vi "Peak tracking sq.vi"(4 "BF len":i32, 6 "EnH choice":u16(ring) items=["Off", "Linear best fit"], 7 "Error control":sgl, 8 "Trace":i32=1, 9 "Poly count":i32=4, 10 "Int IN":sgl[](array[numeric]), 11 "Scan":sgl[][](array[numeric])) -> (2 "Int Out":sgl[](array[numeric]), 3 "Scan Out":sgl[](array[numeric]))   [LabVIEW 2014]
uses:
  <vilib>/Analysis/NI_AALPro.lvlib
panel:
  out "Locations":sgl[](array[numeric])
  # "See block diagram"
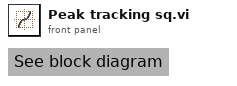
[diagram p1: front panel]
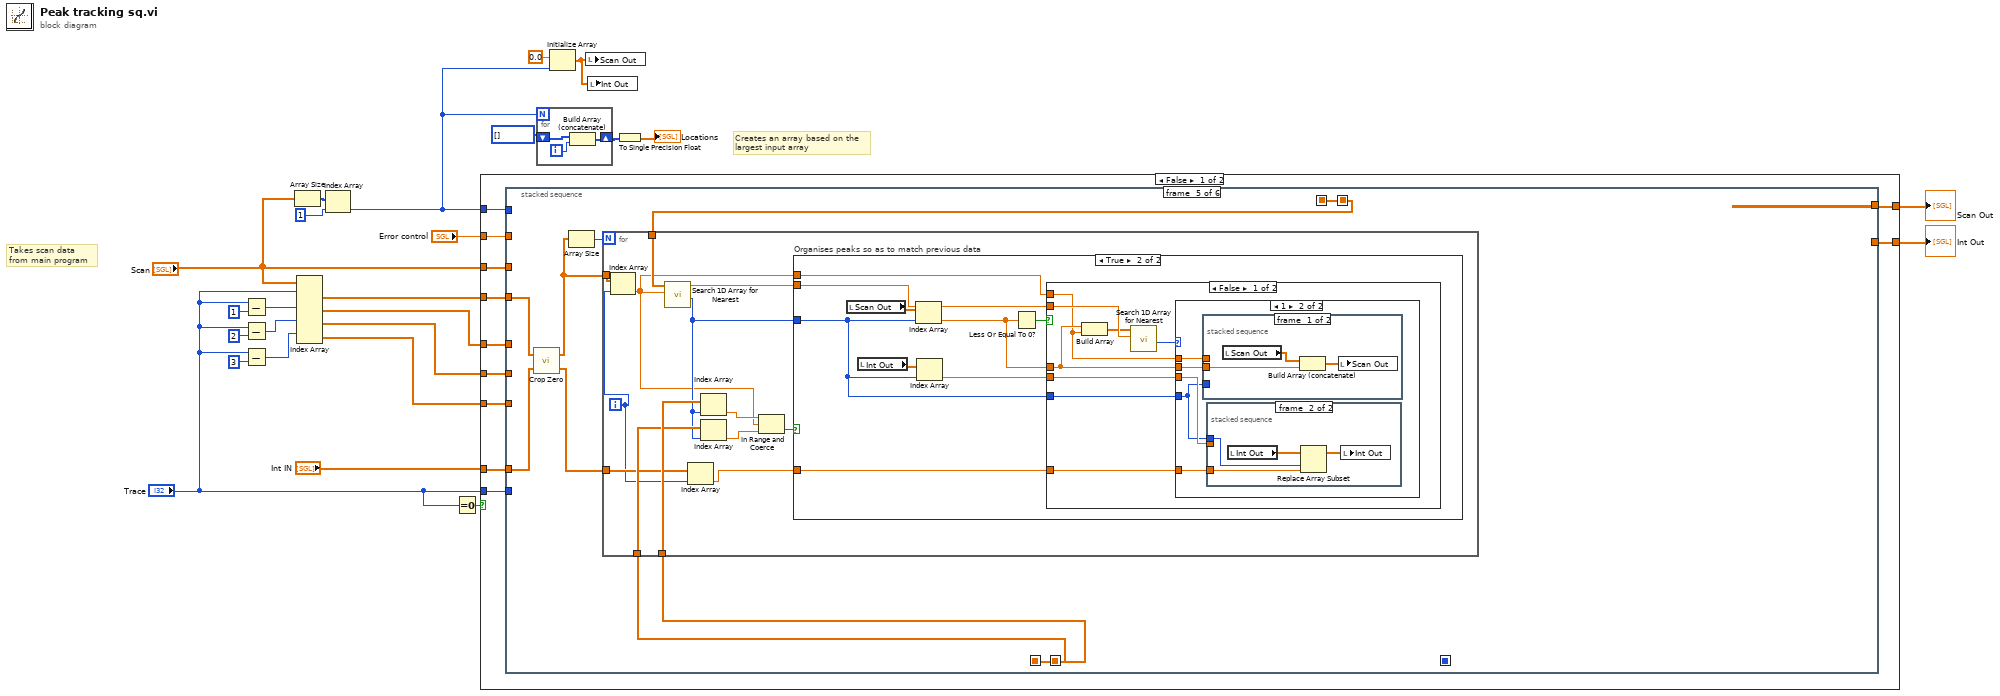
[diagram p0: block diagram]
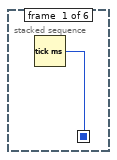
[diagram p2: hidden frame]
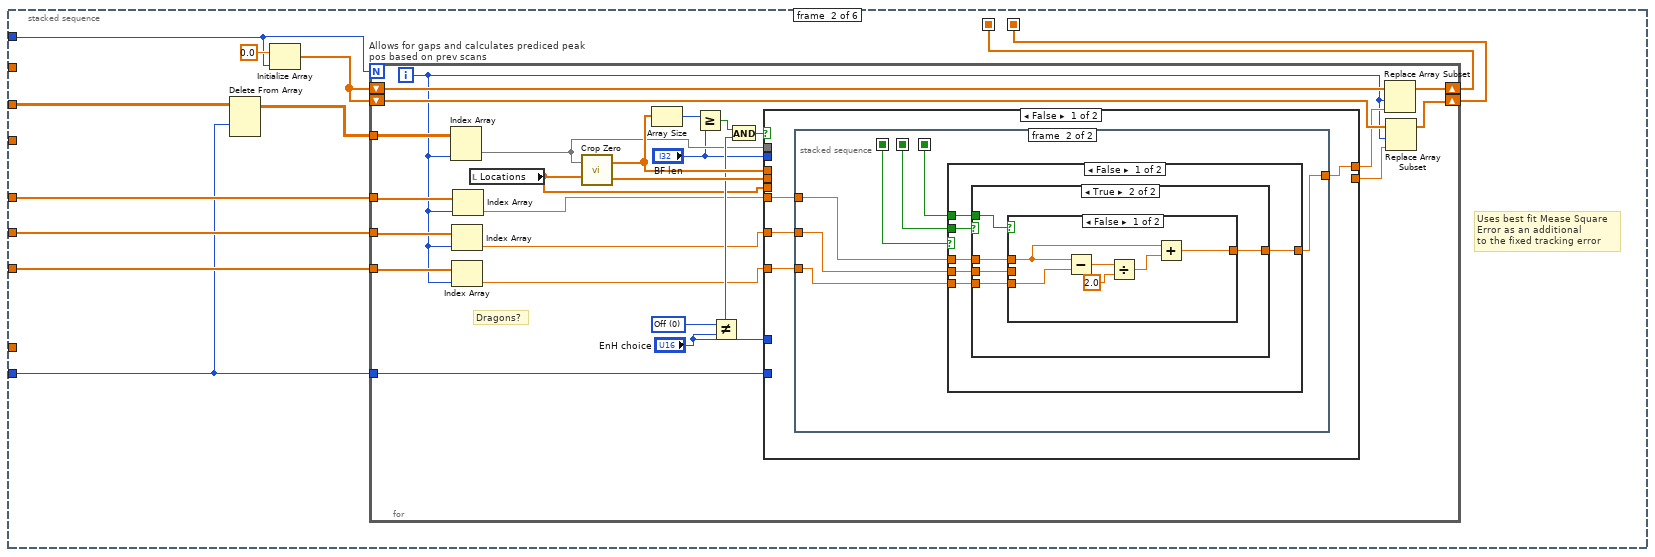
[diagram p3: hidden frame]
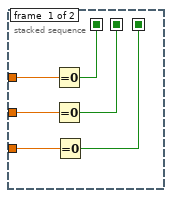
[diagram p4: hidden frame]
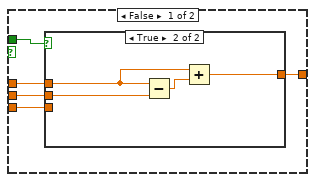
[diagram p5: hidden frame]
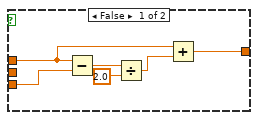
[diagram p6: hidden frame]
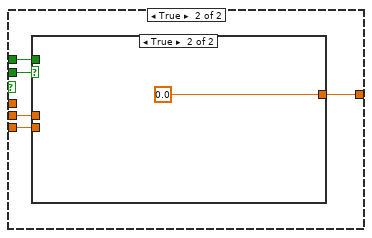
[diagram p8: hidden frame]
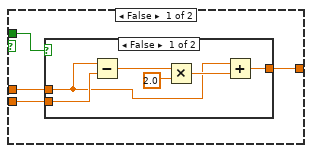
[diagram p9: hidden frame]
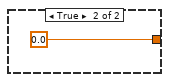
[diagram p10: hidden frame]
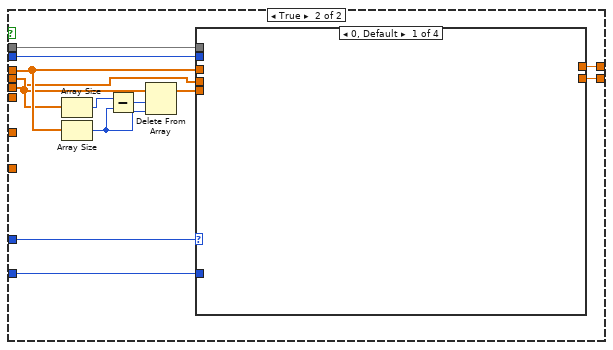
[diagram p11: hidden frame]
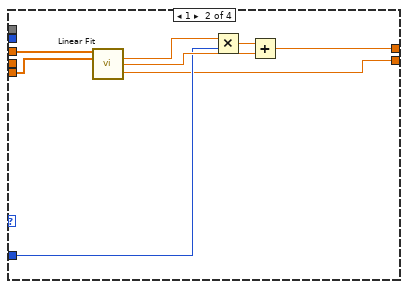
[diagram p12: hidden frame]
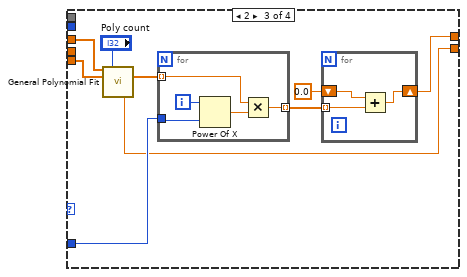
[diagram p13: hidden frame]
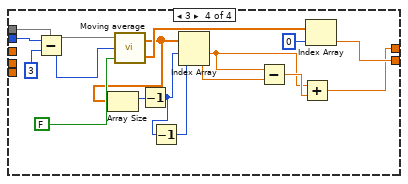
[diagram p14: hidden frame]
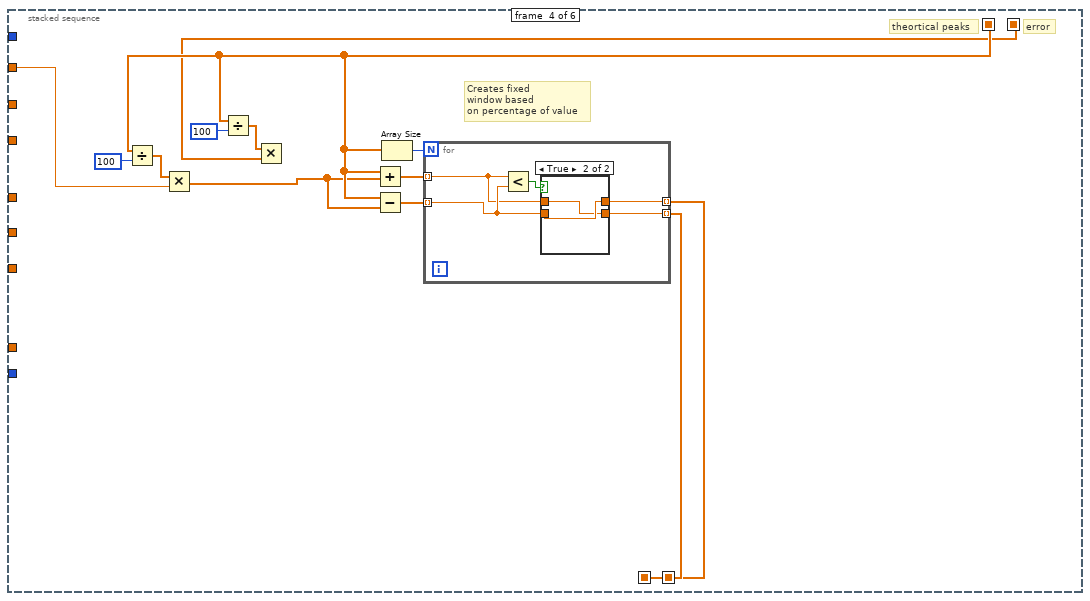
[diagram p16: hidden frame]
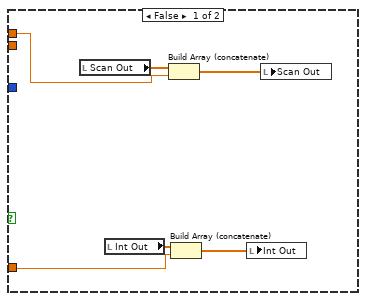
[diagram p18: hidden frame]
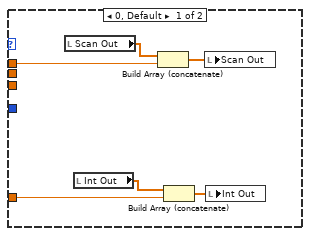
[diagram p19: hidden frame]
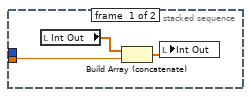
[diagram p20: hidden frame]
diagram:
  # "Takes scan data\nfrom main program"
  # "Creates an array based on the\nlargest input array"
  n1 = Subtract(x="Trace", y=1 ("index (row)")) -> (x-y=w21:i32)
  n2 = Subtract(x="Trace", y=2 ("index (row)")) -> (x-y=w20:i32)
  n3 = Subtract(x="Trace", y=3 ("index (row)")) -> (x-y=w19:i32)
  n4 = Array Size(array="Scan") -> (size(s)=w9:i32[])
  n5 = Index Array(array="Scan", index (row) #1="Trace", index (row) #2=w21, index (row) #3=w20, index (row) #4=w19) -> (element #1=w7:sgl[], element #2=w14:sgl[], element #3=w6:sgl[], element #4=w15:sgl[])  [unwired: 4 in]
  n6 = Index Array(array=w9, index=1) -> (element=w5:i32)
  n7 = Equal To 0?(x="Trace") -> (x = 0?=w3:bool)
  n8 = case shown="False" w3 {
    tunnel: "Error control" -> [w36 _]
    tunnel: [w35 w296] -> w23
    tunnel: w15 -> [w34 _]
    tunnel: w7 -> [w33 w297]
    tunnel: "Int IN" -> [w32 w296]
    tunnel: w14 -> [w31 _]
    tunnel: w6 -> [w30 _]
    tunnel: [w29 w297] -> w13
    tunnel: "Scan" -> [w28 _]
    tunnel: w5 -> [w27 _]
    tunnel: "Trace" -> [w26 _]
    frame False {
      n9 = stacked-sequence {
        seq-local: [_ w46 _ _ _ _] -> [_ _ _ w199 w225 _]
        seq-local: [_ _ _ w208 _ _] -> [_ _ _ _ w224 _]
        seq-local: [_ _ _ w207 _ _] -> [_ _ _ _ w223 _]
        seq-local: [_ w45 _ _ _ _] -> [_ _ _ w198 _ _]
        seq-local: [w37 _ _ _ _ _] -> [_ _ _ _ _ _]
        tunnel: w33 -> [_ _ _ _ w220 _]
        tunnel: w31 -> [_ w43 _ _ _ _]
        tunnel: w30 -> [_ w41 _ _ _ _]
        tunnel: w34 -> [_ w42 _ _ _ _]
        tunnel: w32 -> [_ _ _ _ w222 _]
        tunnel: w36 -> [_ _ _ w206 _ _]
        tunnel: [_ _ _ _ _ w295] -> w29
        tunnel: [_ _ _ _ _ w294] -> w35
        tunnel: w27 -> [_ w38 _ _ _ _]
        tunnel: w28 -> [_ w44 _ _ _ _]
        tunnel: w26 -> [_ w39 _ _ _ _]
        frame #0 {
          n10 = Tick Count (ms)() -> (millisecond timer value=w37:u32)
        }
        frame #1 {
          # "Uses best fit Mease Square\nError as an additional\nto the fixed tracking error"
          n11 = Delete From Array(array=w44, index (row)=w39) -> (array with subset deleted=w40:sgl[][])  [unwired: 2 in, 1 out]
          n12 = Initialize Array(sgl 0.0 ("BLANK"), w38) -> (w48:sgl[])
          n13 = for "Allows for gaps and calculates prediced peak pos based on prev scans" {
            N: w38 -> [_]
            shift-right: [w72] -> w46
            shift-left: w48 -> [w74]
            shift-right: [w71] -> w45
            shift-left: w48 -> [w73]
            tunnel: w40 -> [w53]
            tunnel: w39 -> [w63]
            tunnel: w41 -> [w56]
            tunnel: w43 -> [w55]
            tunnel: w42 -> [w54]
            i -> [w52]
            w62 = u16 0 items=["Off", "Linear best fit"] ("EnH choice")
            # "Dragons?"
            n14 = Index Array(array=w53, index (col)=w52) -> (element=w51:sgl[])  [unwired: 1 in]
            n15 = Index Array(array=w56, index=w52) -> (element=w58:sgl)
            n16 = Index Array(array=w54, index=w52) -> (element=w57:sgl)
            n17 = Index Array(array=w55, index=w52) -> (element=w59:sgl)
            n18 = local read "Locations"() -> (w50:sgl[])
            n19 = call "Crop Zero.vi"("Paired data"=w50, "Search data"=w51) -> ("Paired data out"=w64:sgl[], "Searched data out"=w65:sgl[])
            n20 = Array Size(array=w65) -> (size(s)=w68:i32)
            n21 = Greater Or Equal?(x=w68, y="BF len") -> (x >= y?=w67:bool)
            n22 = Not Equal?(x=w62, y="EnH choice") -> (x != y?=w60:bool)
            n23 = And(x=w67, y=w60) -> (x .and. y?=w66:bool)
            n24 = case shown="False" w66 {
              tunnel: w57 -> [w78 _]
              tunnel: w58 -> [w77 _]
              tunnel: w59 -> [w75 _]
              tunnel: [_ w145] -> w70
              tunnel: [w76 w152] -> w69
              tunnel: "EnH choice" -> [_ w153]
              tunnel: w65 -> [_ w154]
              tunnel: w64 -> [_ w147]
              tunnel: w63 -> [_ w146]
              tunnel: "BF len" -> [_ w144]
              tunnel: w51 -> [_ w143]
              tunnel: w50 -> [_ w142]
              frame False {
                n25 = stacked-sequence {
                  seq-local: [w81 _] -> [_ w88]
                  seq-local: [w80 _] -> [_ w86]
                  seq-local: [w79 _] -> [_ w87]
                  tunnel: w78 -> [w82 w91]
                  tunnel: w77 -> [w83 w90]
                  tunnel: w75 -> [w84 w89]
                  tunnel: [_ w85] -> w76
                  frame #0 {
                    n26 = Equal To 0?(x=w84) -> (x = 0?=w81:bool)
                    n27 = Equal To 0?(x=w83) -> (x = 0?=w80:bool)
                    n28 = Equal To 0?(x=w82) -> (x = 0?=w79:bool)
                  }
                  frame #1 {
                    n29 = case "Is S-1 = 0" shown="False" w88 {
                      tunnel: w91 -> [w97 w126]
                      tunnel: w90 -> [w96 w125]
                      tunnel: w89 -> [w95 _]
                      tunnel: [w94 w127] -> w85
                      tunnel: w86 -> [w92 w129]
                      tunnel: w87 -> [w93 w128]
                      frame False {
                        n30 = case "Is S-2 = 0" shown="True" w92 {
                          tunnel: w97 -> [w102 w117]
                          tunnel: w96 -> [w101 w116]
                          tunnel: w95 -> [w100 w115]
                          tunnel: [w99 w114] -> w94
                          tunnel: w93 -> [w98 w113]
                          frame False {
                            n31 = case "Is S-3 = 0" shown="True" w98 {
                              tunnel: w102 -> [w108 _]
                              tunnel: w101 -> [_ w111]
                              tunnel: w100 -> [w103 w112]
                              tunnel: [w104 w110] -> w99
                              frame False {
                                n32 = Subtract(x=w103, y=w108) -> (x-y=w107:sgl)
                                n33 = Divide(x=w107, y=sgl 2.0) -> (x/y=w105:sgl)
                                n34 = Add(x=w103, y=w105) -> (x+y=w104:sgl)
                              }
                              frame True {
                                n35 = Subtract(x=w112, y=w111) -> (x-y=w109:sgl)
                                n36 = Add(x=w112, y=w109) -> (x+y=w110:sgl)
                              }
                            }
                          }
                          frame True {
                            n37 = case shown="False" w113 {
                              tunnel: w117 -> [w120 _]
                              tunnel: w116 -> [_ _]
                              tunnel: w115 -> [w119 w124]
                              tunnel: [w118 w124] -> w114
                              frame False {
                                n38 = Subtract(x=w119, y=w120) -> (x-y=w121:sgl)
                                n39 = Divide(x=w121, y=sgl 2.0) -> (x/y=w122:sgl)
                                n40 = Add(x=w119, y=w122) -> (x+y=w118:sgl)
                              }
                              frame True {
                              }
                            }
                          }
                        }
                      }
                      frame True {
                        n41 = case "Is S-2 = 0" shown="True" w129 {
                          tunnel: w128 -> [w133 _]
                          tunnel: [w132 sgl 0.0] -> w127
                          tunnel: w126 -> [w131 _]
                          tunnel: w125 -> [w130 _]
                          frame False {
                            n42 = case "Is S-3 = 0" shown="False" w133 {
                              tunnel: [w136 0.0] -> w132
                              tunnel: w131 -> [w135 _]
                              tunnel: w130 -> [w134 _]
                              frame False {
                                n43 = Subtract(x=w134, y=w135) -> (x-y=w137:sgl)
                                n44 = Multiply(x=w137, y=sgl 2.0) -> (x*y=w138:sgl)
                                n45 = Add(x=w134, y=w138) -> (x+y=w136:sgl)
                              }
                              frame True {
                              }
                            }
                          }
                          frame True {
                          }
                        }
                      }
                    }
                  }
                }
              }
              frame True {
                n46 = Array Size(array=w147) -> (size(s)=w149:i32)
                n47 = Array Size(array=w154) -> (size(s)=w150:i32)
                n48 = Subtract(x=w149, y=w150) -> (x-y=w151:i32)
                n49 = Delete From Array(array=w147, length=w151, index=w150) -> (array with subset deleted=w148:sgl[])  [unwired: 1 out]
                n50 = case shown="0, Default" w153 {
                  tunnel: w154 -> [_ w157 w171 _]
                  tunnel: w148 -> [_ w158 w170 _]
                  tunnel: [_ w159 w165 w188] -> w152
                  tunnel: w146 -> [_ w156 w166 _]
                  tunnel: [_ w155 w163 w193] -> w145
                  tunnel: w144 -> [_ _ _ w182]
                  tunnel: w143 -> [_ _ _ w195]
                  tunnel: w142 -> [_ _ _ _]
                  frame 0, Default {
                  }
                  frame 1 {
                    n51 = call <vilib>:"Linear Fit.vi"("Y"=w157, "X"=w158) -> ("slope"=w162:dbl, "intercept"=w161:dbl, "residue"=w155:dbl)  [unwired: 9 in, 2 out]
                    n52 = Multiply(x=w162, y=w156) -> (x*y=w160:dbl)
                    n53 = Add(x=w160, y=w161) -> (x+y=w159:dbl)
                  }
                  frame 2 {
                    n54 = call <vilib>:"General Polynomial Fit.vi"("Y"=w171, "polynomial order"="Poly count", "X"=w170) -> ("Polynomial Coefficients"=w167:dbl[], "residue"=w163:dbl)  [unwired: 9 in, 2 out]
                    n55 = for {
                      tunnel: w166 -> [w178]
                      tunnel: w167 -> [w175] mode=indexing
                      tunnel: [w176] -> w168 mode=indexing
                      i -> [w179]
                      n56 = Power Of X(1:w178, 2:w179) -> (0:w177:dbl)
                      n57 = Multiply(x=w175, y=w177) -> (x*y=w176:dbl)
                    }
                    n58 = for {
                      tunnel: w168 -> [w174] mode=indexing
                      shift-right: [w172] -> w165
                      shift-left: 0.0 -> [w173]
                      n59 = Add(x=w173, y=w174) -> (x+y=w172:dbl)
                    }
                  }
                  frame 3 {
                    n60 = Subtract(x=w182, y=3) -> (x-y=w181:i32)
                    n61 = call "Moving average.vi"("Central mAV t/f (t)"=FALSE, "Width of AV"=w181, "Raw data"=w195) -> ("Data STDEVs"=w194:dbl[], "Data AVs"=w186:dbl[])
                    n62 = Array Size(array=w186) -> (size(s)=w185:i32)
                    n63 = Decrement(x=w185) -> (x-1=w184:i32)
                    n64 = Decrement(x=w184) -> (x-1=w183:i32)
                    n65 = Index Array(array=w186, index #1=w184, index #2=w183) -> (element #1=w189:dbl, element #2=w191:dbl)
                    n66 = Subtract(x=w189, y=w191) -> (x-y=w190:dbl)
                    n67 = Add(x=w189, y=w190) -> (x+y=w188:dbl)
                    n68 = Index Array(array=w194, index=0) -> (element=w193:dbl)
                  }
                }
              }
            }
            n69 = Replace Array Subset(array=w74, new element=w69, index=w52) -> (w72:sgl[])
            n70 = Replace Array Subset(array=w73, new element=w70, index=w52) -> (w71:sgl[])
          }
        }
        frame #2 {
        }
        frame #3 {
          # "error"
          # "theortical peaks"
          # "Creates fixed\nwindow based \non percentage of value"
          n71 = Divide(x=w199, y=100) -> (x/y=w201:sgl[])
          n72 = Multiply(x=w201, y=w206) -> (x*y=w196:sgl[])
          n73 = Divide(x=w199, y=100) -> (x/y=w197:sgl[])
          n74 = Multiply(x=w197, y=w198) -> ()  [unwired: 1 out]
          n75 = Add(x=w199, y=w196) -> (x+y=w205:sgl[])
          n76 = Subtract(x=w199, y=w196) -> (x-y=w203:sgl[])
          n77 = Array Size(array=w199) -> (size(s)=w204:i32)
          n78 = for {
            N: w204 -> [_]
            tunnel: w205 -> [w210] mode=indexing
            tunnel: w203 -> [w212] mode=indexing
            tunnel: [w209] -> w207 mode=indexing
            tunnel: [w213] -> w208 mode=indexing
            n79 = Less?(x=w210, y=w212) -> (x < y?=w211:bool)
            n80 = case shown="True" w211 {
              tunnel: w210 -> [w215 w216]
              tunnel: w212 -> [w214 w217]
              tunnel: [w215 w217] -> w209
              tunnel: [w214 w216] -> w213
              frame False {
              }
              frame True {
              }
            }
          }
        }
        frame #4 {
          n81 = call "Crop Zero.vi"("Paired data"=w222, "Search data"=w220) -> ("Paired data out"=w221:sgl[], "Searched data out"=w218:sgl[])
          n82 = Array Size(array=w218) -> (size(s)=w219:i32)
          n83 = for {
            N: w219 -> [_]
            tunnel: w218 -> [w229]
            tunnel: w225 -> [w238]
            tunnel: w224 -> [w234]
            tunnel: w223 -> [w236]
            tunnel: w221 -> [w227]
            i -> [w226]
            n84 = Index Array(array=w229, index=w226) -> (element=w230:sgl)
            n85 = call "Search 1D Array for Nearest.vi"("desired element"=w230, "1D Array"=w238) -> ("closest index"=w231:i32, "closest element"=w233:dbl)  [unwired: 8 in]
            n86 = Index Array(array=w227, index=w226) -> (element=w228:sgl)
            n87 = Index Array(array=w236, index=w231) -> (element=w237:sgl)
            n88 = Index Array(array=w234, index=w231) -> (element=w235:sgl)
            n89 = In Range and Coerce(upper limit=w237, x=w230, lower limit=w235) -> (In Range?=w232:bool)  [unwired: 1 out]
            n90 = case "Organises peaks so as to match previous data" shown="True" w232 {
              tunnel: w231 -> [_ w245]
              tunnel: w230 -> [w244 w253]
              tunnel: w228 -> [w243 w248]
              tunnel: w233 -> [_ w249]
              frame False {
                n91 = local read "Scan Out"() -> (w240:sgl[])
                n92 = local read "Int Out"() -> (w241:sgl[])
                n93 = Build Array (concatenate)(w240, w244) -> (w239:sgl[])
                n94 = Build Array (concatenate)(w241, w243) -> (w242:sgl[])
                n95 = local write "Int Out"(w242) -> ()
                n96 = local write "Scan Out"(w239) -> ()
              }
              frame True {
                n97 = local read "Scan Out"() -> (w252:sgl[])
                n98 = local read "Int Out"() -> (w247:sgl[])
                n99 = Index Array(array=w252, index=w245) -> (element=w250:sgl)
                n100 = Index Array(array=w247, index=w245) -> (element=w246:sgl)
                n101 = Less Or Equal To 0?(x=w250) -> (x <= 0?=w251:bool)
                n102 = case "If two values match t" shown="False" w251 {
                  tunnel: w253 -> [w254 w293]
                  tunnel: w245 -> [w255 w292]
                  tunnel: w250 -> [w257 _]
                  tunnel: w249 -> [w261 _]
                  tunnel: w248 -> [w258 w291]
                  tunnel: w246 -> [w256 _]
                  frame False {
                    n103 = Build Array(w257, w254) -> (w260:sgl[])
                    n104 = call "Search 1D Array for Nearest.vi"("desired element"=w261, "1D Array"=w260) -> ("closest index"=w259:i32)  [unwired: 8 in, 1 out]
                    n105 = case shown="1" w259 {
                      tunnel: w254 -> [w263 w269]
                      tunnel: w258 -> [w262 w272]
                      tunnel: w257 -> [_ w270]
                      tunnel: w256 -> [_ w271]
                      tunnel: w255 -> [_ w268]
                      frame 0, Default {
                        n106 = local read "Scan Out"() -> (w267:sgl[])
                        n107 = local read "Int Out"() -> (w265:sgl[])
                        n108 = Build Array (concatenate)(w267, w263) -> (w266:sgl[])
                        n109 = Build Array (concatenate)(w265, w262) -> (w264:sgl[])
                        n110 = local write "Scan Out"(w266) -> ()
                        n111 = local write "Int Out"(w264) -> ()
                      }
                      frame 1 {
                        n112 = stacked-sequence {
                          tunnel: w268 -> [_ w285]
                          tunnel: w270 -> [w281 _]
                          tunnel: w269 -> [_ w284]
                          frame #0 {
                            n113 = local read "Scan Out"() -> (w280:sgl[])
                            n114 = Build Array (concatenate)(w280, w281) -> (w282:sgl[])
                            n115 = local write "Scan Out"(w282) -> ()
                          }
                          frame #1 {
                            n116 = local read "Scan Out"() -> (w283:sgl[])
                            n117 = Replace Array Subset(array=w283, new element=w284, index=w285) -> (w286:sgl[])
                            n118 = local write "Scan Out"(w286) -> ()
                          }
                        }
                        n119 = stacked-sequence {
                          tunnel: w272 -> [_ w277]
                          tunnel: w271 -> [w273 _]
                          tunnel: w268 -> [_ w276]
                          frame #0 {
                            n120 = local read "Int Out"() -> (w274:sgl[])
                            n121 = Build Array (concatenate)(w274, w273) -> (w275:sgl[])
                            n122 = local write "Int Out"(w275) -> ()
                          }
                          frame #1 {
                            n123 = local read "Int Out"() -> (w278:sgl[])
                            n124 = Replace Array Subset(array=w278, new element=w277, index=w276) -> (w279:sgl[])
                            n125 = local write "Int Out"(w279) -> ()
                          }
                        }
                      }
                    }
                  }
                  frame True {
                    n126 = local read "Scan Out"() -> (w289:sgl[])
                    n127 = local read "Int Out"() -> (w288:sgl[])
                    n128 = Replace Array Subset(array=w289, new element=w293, index=w292) -> (w290:sgl[])
                    n129 = Replace Array Subset(array=w288, new element=w291, index=w292) -> (w287:sgl[])
                    n130 = local write "Scan Out"(w290) -> ()
                    n131 = local write "Int Out"(w287) -> ()
                  }
                }
              }
            }
          }
        }
        frame #5 {
          # "Sends final organised data\nback to peak tracking software"
          n132 = local read "Scan Out"() -> (w295:sgl[])
          n133 = local read "Int Out"() -> (w294:sgl[])
        }
      }
    }
    frame True {
    }
  }
  "Scan Out" <- w13
  "Int Out" <- w23
  n134 = for {
    N: w5 -> [_]
    shift-right: [w299] -> w11
    shift-left: i32[] [] -> [w300]
    i -> [w298]
    n135 = Build Array (concatenate)(w300, w298) -> (w299:i32[])
  }
  n136 = Initialize Array(sgl 0.0 ("BLANK"), w5) -> (w22:sgl[])
  n137 = local write "Scan Out"(w22) -> ()
  n138 = local write "Int Out"(w22) -> ()
  n139 = To Single Precision Float(number=w11) -> (single precision float=→"Locations":sgl[])
